vi "CreateExecuteCommand.vi"   [LabVIEW 2017]
uses:
  <vilib>/Utility/miscctls.llb/LVPointTypeDef.ctl
types:
  T1 = enum32{"Invalid", "Standard", "Closed", "Hidden", "Minimized", "Maximized"}
  T2 = typedef "LVPointTypeDef.ctl" = cluster{"Horizontal":i16, "Vertical":i16}
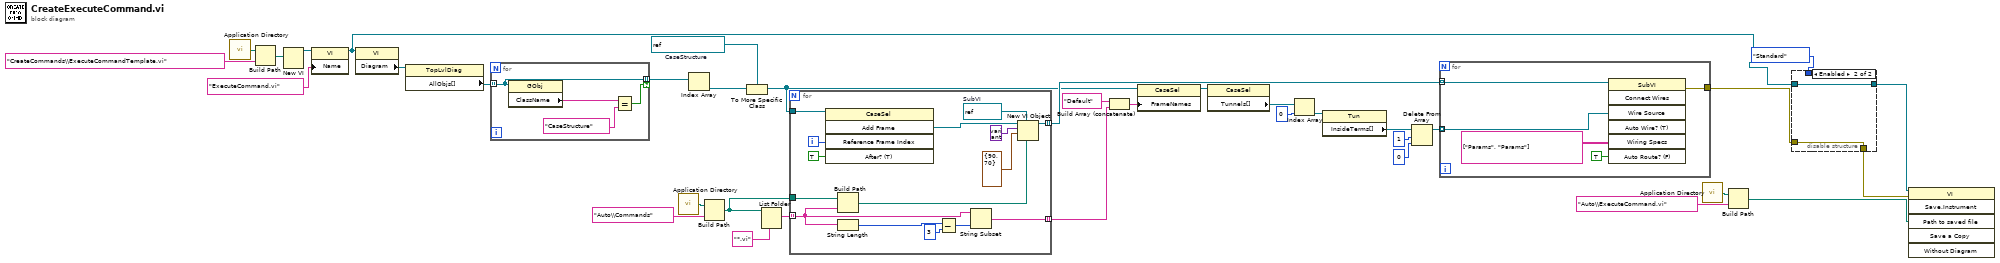
[diagram p0: block diagram]
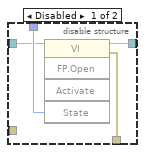
[diagram p2: hidden frame]
diagram:
  w32 = refnum<vi> refnum  # CaseStructure
  n1 = call <vilib>:"Application Directory.vi"() -> ("Application Directory"=w14:path)
  n2 = Build Path(base path=w14, name or relative path="CreateCommands\\ExecuteCommandTemplate.vi") -> (appended path=w12:path)
  n3 = New VI(10:w12) -> (3:w36:refnum<vi>)  [unwired: 6 in, 1 out]
  n4 = property class="VI"(reference=w36, "Name"="ExecuteCommand.vi" ("VI Name")) -> (reference out=w5:refnum<vi>)  [unwired: 1 in, 1 out]
  n5 = property class="VI"(reference=w5) -> ("Diagram"=w35:refnum<vi>)  [unwired: 1 in, 2 out]
  n6 = property class="TopLvlDiag"(reference=w35) -> ("AllObjs[]"=w25:refnum<vi>[])  [unwired: 1 in, 2 out]
  n7 = for {
    tunnel: w25 -> [w37] mode=indexing
    tunnel: [w37] -> w34 mode=indexing if=w38
    n8 = property class="GObj"(reference=w37) -> ("ClassName"=w40:string)  [unwired: 1 in, 2 out]
    n9 = Equal?(x=w40, y="CaseStructure") -> (x = y?=w38:bool)
  }
  n10 = call <vilib>:"Application Directory.vi"() -> ("Application Directory"=w10:path)
  n11 = Index Array(array=w34) -> (element=w33:refnum<vi>)  [unwired: 1 in]
  n12 = Build Path(base path=w10, name or relative path="Auto\\Commands") -> (appended path=w9:path)
  n13 = To More Specific Class(target class=w32, reference=w33) -> (specific class reference=w15:refnum<vi>)  [unwired: 1 in, 1 out]
  n14 = List Folder(path=w9, pattern="*.vi") -> (filenames=w30:string[])  [unwired: 2 in, 3 out]
  n15 = for {
    tunnel: w15 -> [w54]
    tunnel: w30 -> [w45] mode=indexing
    tunnel: [w41] -> w29 mode=indexing
    tunnel: w9 -> [w53]
    tunnel: [w46] -> w21 mode=indexing
    i -> [w48]
    w51 = refnum<vi> refnum  # SubVI
    n16 = invoke class="CaseSel" method="Add Frame"(reference=w54, "Reference Frame Index"=w48, "After? (T)"=TRUE) -> ("Add Frame"=w47:refnum<vi>)  [unwired: 2 in, 4 out]
    n17 = Build Path(base path=w53, name or relative path=w45) -> (appended path=w52:path)
    n18 = String Length(string=w45) -> (length=w44:i32)
    n19 = Subtract(x=w44, y=3) -> (x-y=w42:i32)
    n20 = String Subset(string=w45, length (rest)=w42) -> (substring=w41:string)  [unwired: 1 in]
    n21 = New VI Object(vi object class=w51, owner refnum=w47, style=variant, position/next to=T2 {"Horizontal"=90, "Vertical"=70} ("location"), 6:w52) -> (object refnum=w46:refnum<vi>)  [unwired: 3 in, 1 out]
  }
  n22 = Build Array (concatenate)("Default", w29) -> (w28:string[])
  n23 = property class="CaseSel"(reference=w15, "FrameNames"=w28) -> (reference out=w20:refnum<vi>)  [unwired: 1 in, 1 out]
  n24 = property class="CaseSel"(reference=w20) -> ("Tunnels[]"=w22:refnum<vi>[])  [unwired: 1 in, 2 out]
  n25 = Index Array(array=w22, index=0) -> (element=w23:refnum<vi>)
  n26 = property class="Tun"(reference=w23) -> ("InsideTerms[]"=w19:refnum<vi>[])  [unwired: 1 in, 2 out]
  n27 = Delete From Array(array=w19, length=1, index=0) -> (array with subset deleted=w16:refnum<vi>[])  [unwired: 1 out]
  n28 = for {
    tunnel: w21 -> [w60] mode=indexing
    tunnel: w16 -> [w57] mode=indexing
    tunnel: [w56] -> w1
    n29 = invoke class="SubVI" method="Connect Wires"(reference=w60, "Wire Source"=w57, "Wiring Specs"=string[][] [["Params", "Params"]], "Auto Route? (F)"=TRUE) -> (error out=w56:errorcluster)  [unwired: 3 in, 6 out]
  }
  n30 = call <vilib>:"Application Directory.vi"() -> ("Application Directory"=w8:path)
  n31 = Build Path(base path=w8, name or relative path="Auto\\ExecuteCommand.vi") -> (appended path=w3:path)
  n32 = disable-structure shown="Enabled" {
    disable-tunnel: T1."Standard" ("State") -> [w64 _]
    disable-tunnel: w5 -> [w63 w66]
    disable-tunnel: [w62 w66] -> w4
    disable-tunnel: [w61 w65] -> w2
    disable-tunnel: w1 -> [_ w65]
    frame Disabled {
      n33 = invoke class="VI" method="FP.Open"(reference=w63, "State"=w64) -> (reference out=w62:refnum<vi>, error out=w61:errorcluster)  [unwired: 3 in, 3 out]
    }
    frame Enabled {
    }
  }
  n34 = invoke class="VI" method="Save.Instrument"(reference=w4, error in=w2, "Path to saved file"=w3) -> ()  [unwired: 3 in, 6 out]
